vi "3DS Rotate and Scale Model.vi"(8 "error in (no error)":errorcluster, 9 "scale":sgl=1.0, 10 "point3f - SHIFT":T2 {"z" format="%.2f"; "y" format="%.2f"; "x" format="%.2f"}, 11 "Object In":T1 {"NormalList"."z" format="%.2f"; "NormalList"."y" format="%.2f"; "NormalList"."x" format="%.2f"; "VertexList"."z" format="%.2f"; "VertexList"."y" format="%.2f"; "VertexList"."x" format="%.2f"}) -> (0 "error out (dup)":errorcluster, 4 "Object Out":T1={"VertexList"=[], "FaceList"=[], "NormalList"=[], "Mode"=enum."GL_TRIANGLES"} {"NormalList"."z" format="%.2f"; "NormalList"."y" format="%.2f"; "NormalList"."x" format="%.2f"; "VertexList"."z" format="%.2f"; "VertexList"."y" format="%.2f"; "VertexList"."x" format="%.2f"}, 5 "FaceList":cluster{"v1":i32, "v2":i32, "v3":i32}[](array[cluster]), 7 "Vertex":T2[](array[typedef]) {"z" format="%.2f"; "y" format="%.2f"; "x" format="%.2f"})   [LabVIEW 2026, in "3D utilities.lvlib"]
uses:
  3D utilities.lvlib
  <vilib>/picture/3D Picture Control/Old 3D Toolkit.llb/model.ctl
  <vilib>/picture/3D Picture Control/Old 3D Toolkit.llb/point3f.ctl
  <vilib>/picture/3D Picture Control/Old 3D Toolkit.llb/VertexMode.ctl
  <vilib>/picture/3D Picture Control/NI_Old 3D Toolkit.lvlib
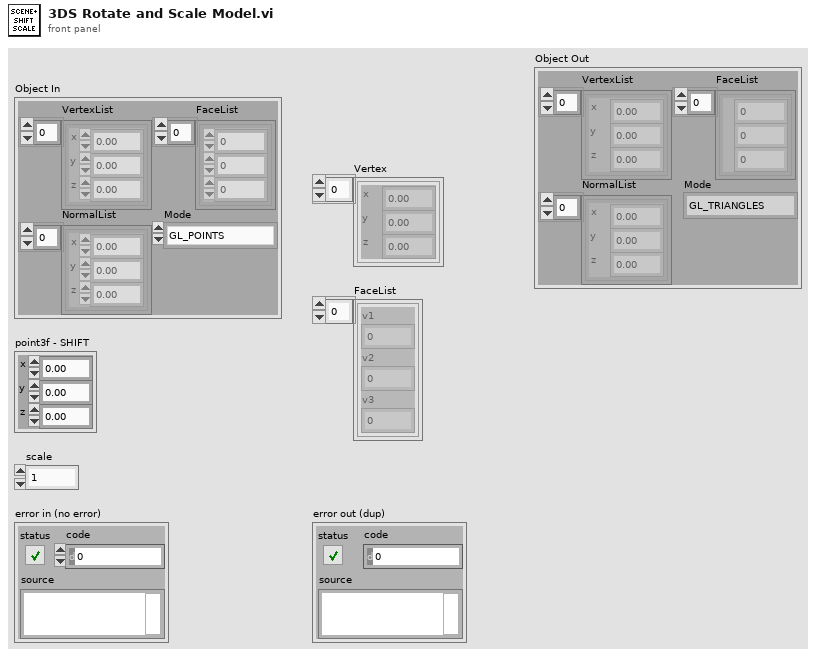
[diagram p1: front panel]
types:
  T1 = typedef "NI_3D Picture Control.lvlib/NI_Old 3D Toolkit.lvlib/model.ctl" = cluster{"VertexList":T2[], "FaceList":cluster{"v1":i32, "v2":i32, "v3":i32}[], "NormalList":T2[], "Mode":T3}
  T2 = typedef "NI_3D Picture Control.lvlib/NI_Old 3D Toolkit.lvlib/point3f.ctl" = cluster{"x":sgl, "y":sgl, "z":sgl}
  T3 = typedef "NI_3D Picture Control.lvlib/NI_Old 3D Toolkit.lvlib/VertexMode.ctl" = enum16{"GL_POINTS", "GL_LINES", "GL_LINE_LOOP", "GL_LINE_STRIP", "GL_TRIANGLES", "GL_TRIANGLE_STRIP", "GL_TRIANGLE_FAN", "GL_QUADS", "GL_QUAD_STRIP", "GL_POLYGON"}
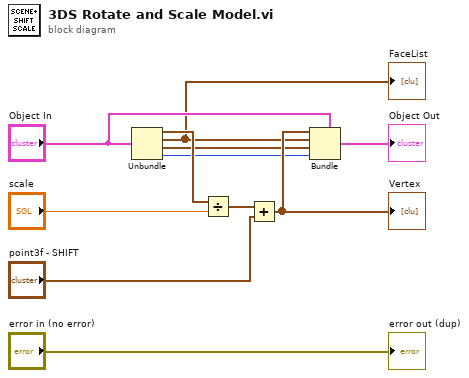
[diagram p0: block diagram]
diagram:
  n1 = Unbundle("Object In") -> ("VertexList"=w10:T2[], "FaceList"=w5:cluster{"v1":i32, "v2":i32, "v3":i32}[], "NormalList"=w4:T2[], "Mode"=w3:T3)
  "FaceList" <- w5
  n2 = Divide(x=w10, y="scale") -> (x/y=w11:T2[])
  n3 = Add(x=w11, y="point3f - SHIFT") -> (x+y=w6:T2[])
  "Vertex" <- w6
  n4 = Bundle(cluster="Object In", "VertexList"=w6, "FaceList"=w5, "NormalList"=w4, "Mode"=w3) -> (→"Object Out":T1)
  "error out (dup)" <- "error in (no error)"
